vi "step6 DoSequence.vi"(11 "cube in":T1) -> (3 "cube out":T1)   [LabVIEW 2011]
uses:
  Typedef/cube.ctl
  Typedef/face.ctl
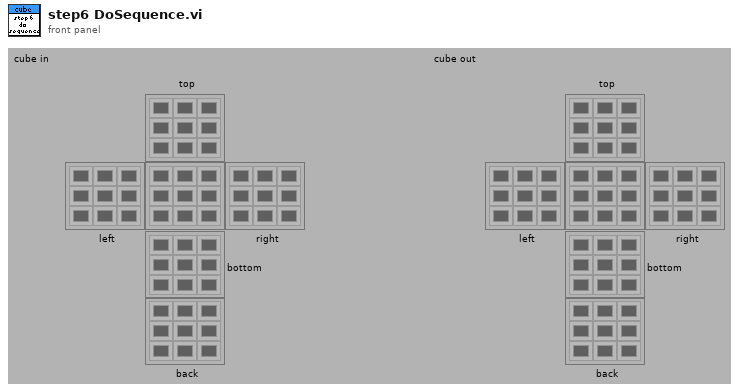
[diagram p1: front panel]
types:
  T1 = typedef "cube.ctl" = cluster{"top":T2, "left":T2, "right":T2, "bottom":T2, "back":T2, "front":T2}
  T2 = typedef "face.ctl" = u32[][]
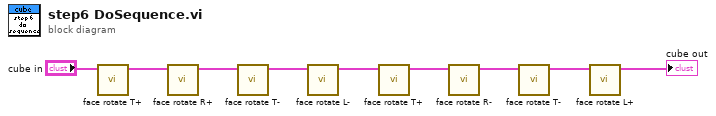
[diagram p0: block diagram]
diagram:
  n1 = call "face rotate T+.vi"("cube in"="cube in") -> ("cube out"=w2:T1)  [unwired: 9 in, 1 out]
  n2 = call "face rotate R+.vi"("cube in"=w2) -> ("cube out"=w3:T1)  [unwired: 9 in, 1 out]
  n3 = call "face rotate T-.vi"("cube in"=w3) -> ("cube out"=w4:T1)  [unwired: 9 in, 1 out]
  n4 = call "face rotate L-.vi"("cube in"=w4) -> ("cube out"=w5:T1)  [unwired: 9 in, 1 out]
  n5 = call "face rotate T+.vi"("cube in"=w5) -> ("cube out"=w6:T1)  [unwired: 9 in, 1 out]
  n6 = call "face rotate R-.vi"("cube in"=w6) -> ("cube out"=w7:T1)  [unwired: 9 in, 1 out]
  n7 = call "face rotate T-.vi"("cube in"=w7) -> ("cube out"=w8:T1)  [unwired: 9 in, 1 out]
  n8 = call "face rotate L+.vi"("cube in"=w8) -> ("cube out"=→"cube out":T1)  [unwired: 9 in, 1 out]
